vi "SENS_PATH_CONF_SEL.vi"(0 "VISA IN":refnum<visa-resource-name>, 3 "FileName":string, 5 "error in":errorcluster, 7 "Channel":i32) -> (14 "VISA Out":refnum<visa-resource-name>, 19 "error out":errorcluster)   [LabVIEW 2018, in "PNA-X.lvlib"]
doc: "SENSe:PATH:CONFiguration:DELete <string>\n(Write-only) Deletes the specified configuration name from the PNA. The factory configurations cannot be deleted. This is the only method of distinguishing a factory configuration from a user-named configuration.\n \nParameters\n \n \n<string>\n Configuration name to be deleted.\n \nExamples\n SENS:PATH:CONF:DEL \"MyMixer\"\n \nReturn Type\n Not Applicable\n \nDefault\n Not Applicable"
uses:
  PNA-X.lvlib
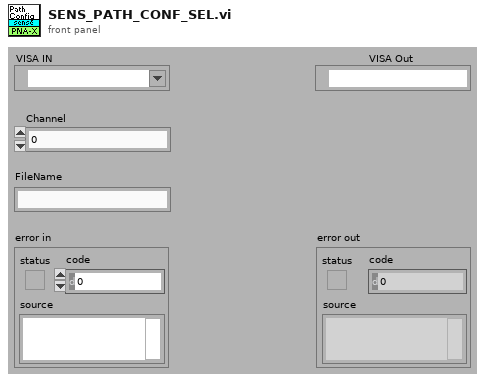
[diagram p1: front panel]
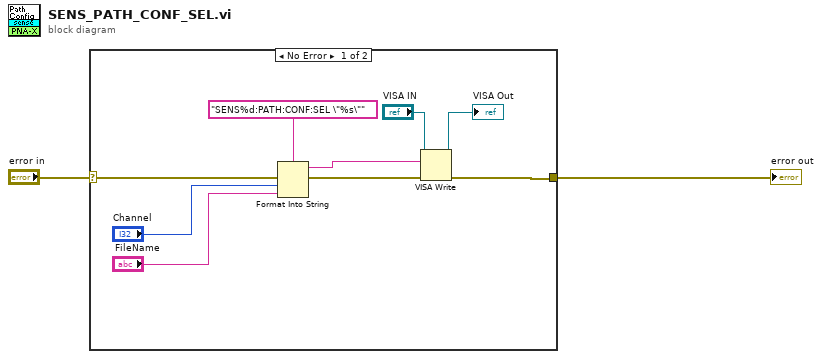
[diagram p0: block diagram]
diagram:
  n1 = case shown="No Error" "error in" {
    selector: "error in" -> [w9 w12]
    tunnel: [w6 w12] -> w1
    frame No Error {
      n2 = Format Into String(format string="SENS%d:PATH:CONF:SEL \"%s\"" ("Cmdline"), error in=w9, "Channel", "FileName") -> (resulting string=w8:string, error out=w10:errorcluster)  [unwired: 1 in]
      n3 = VISA Write(VISA resource name="VISA IN", write buffer=w8, error in (no error)=w10) -> (VISA resource name out=→"VISA Out":refnum<visa-resource-name>, error out=w6:errorcluster)  [unwired: 1 out]
    }
    frame Error {
    }
  }
  "error out" <- w1
